vi "FindCircleCenter.vi"(7 "error in":errorcluster) -> (27 "error out":errorcluster)   [LabVIEW 2017]
uses:
  <vilib>/gmath/GlobalOptimization.llb/DE_State.ctl
  <vilib>/gmath/GlobalOptimization.llb/DE_Population.ctl
  <vilib>/vision/NI_Vision_Development_Module.lvlib
  <vilib>/gmath/NI_AAL_GlobalOptimization.lvlib
panel:
  out "Ending State":T1
  out "XY Graph - Dark":cluster{i32[], dbl[]}[](graph) caption="XY Graph - dark"
  out "Image Out":T3(plugin-control)
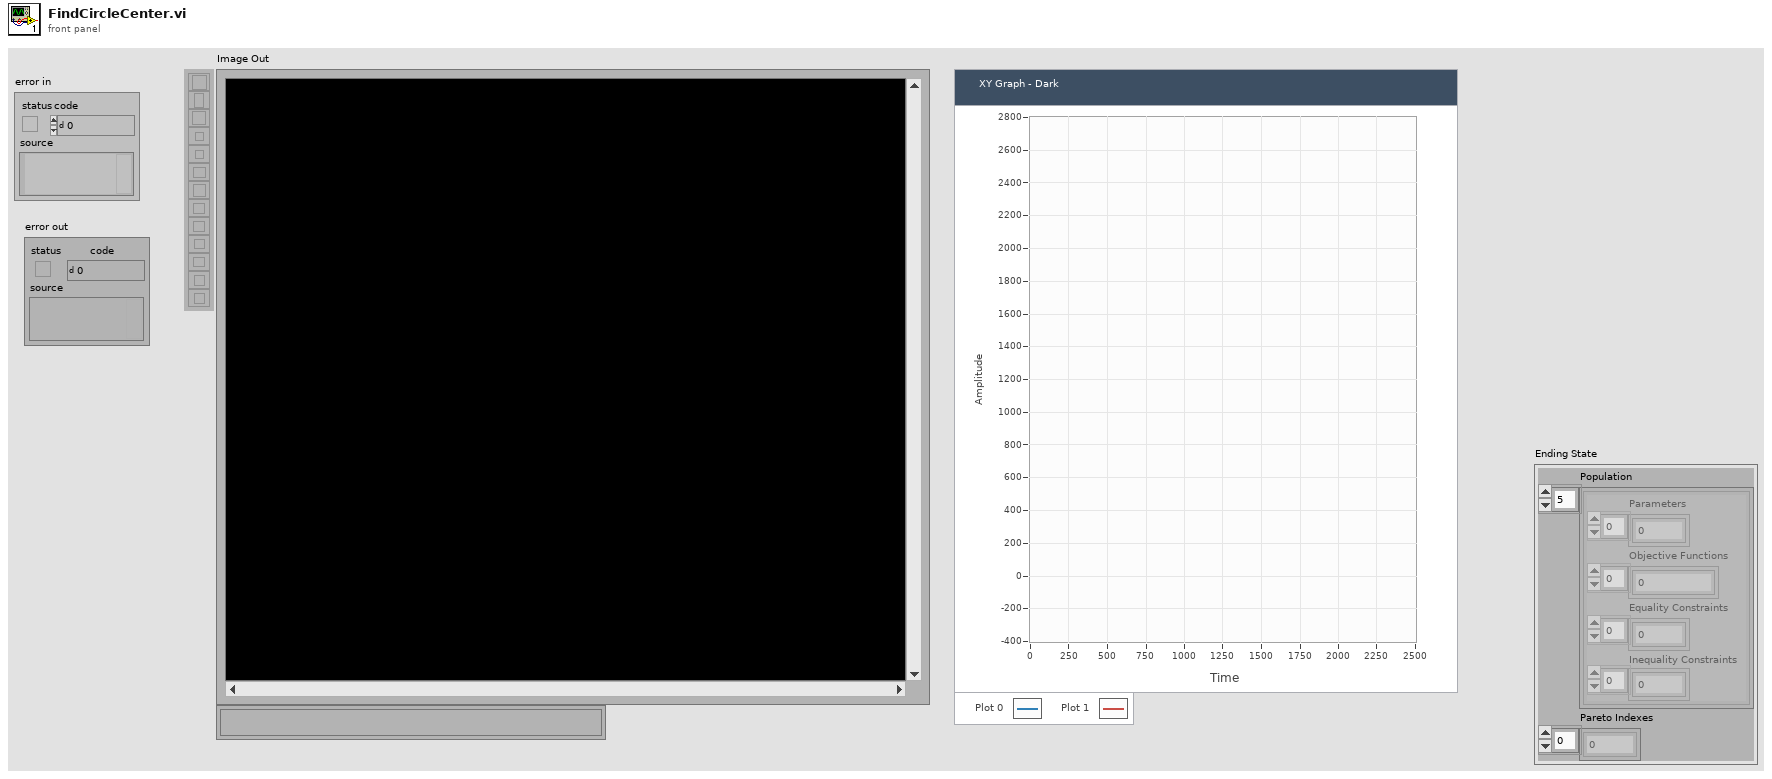
[diagram p1: front panel]
types:
  T1 = typedef "NI_AAL_GlobalOptimization.lvlib/DE_State.ctl" = cluster{"Population":T2[], "Pareto Indexes":i32[]}
  T2 = typedef "NI_AAL_GlobalOptimization.lvlib/DE_Population.ctl" = cluster{"Parameters":dbl[], "Objective Functions":dbl[], "Equality Constraints":dbl[], "Inequality Constraints":dbl[]}
  T3 = typedef "IMAQ Image.ctl" = refnum<image>
  T4 = enum32{"Differentiation", "Gradient", "Prewitt", "Roberts", "Sigma", "Sobel"}
  T5 = typedef "Image Type" = u32
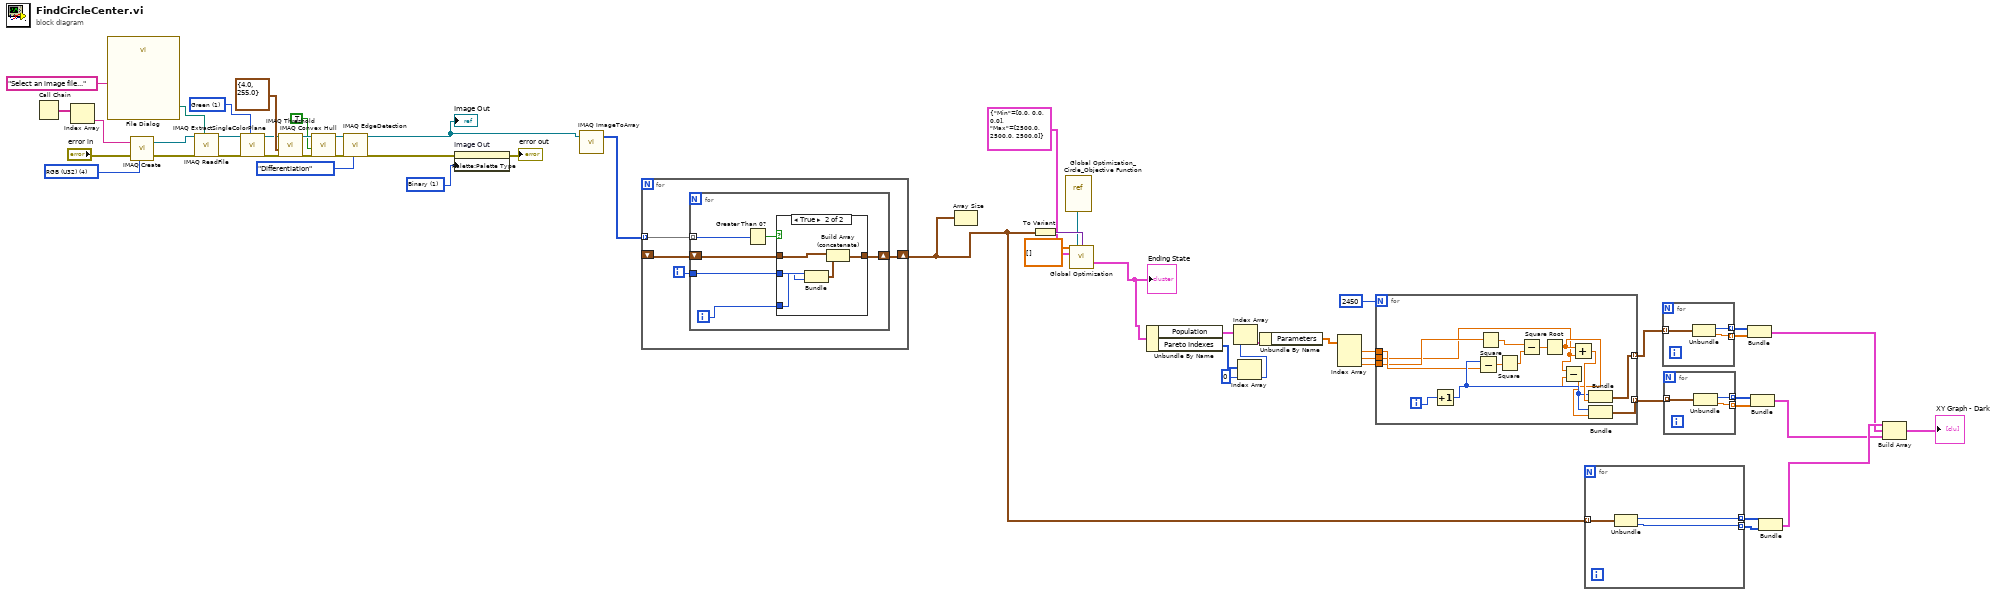
[diagram p0: block diagram]
diagram:
  w31 = u32 1 items=["Grayscale", "Binary", "Gradient", "Rainbow", "Temperature", "User Defined", "Binary 16 Bit", "Gradient 16 Bit", "Rainbow 16 Bit", "Temperature 16 Bit", "User Defined 16 Bit"] ("Palette Type")
  w45 = 1 items=["Red", "Green", "Blue", "Hue", "Saturation", "Luminance", "Value", "Intensity"] ("Color Plane")
  w46 = T5 4 items=["Grayscale (U8)", "Grayscale (I16)", "Grayscale (SGL)", "Complex (CSG)", "RGB (U32)", "HSL (U32)", "RGB (U64)", "Grayscale (U16)"] ("Image Type")
  n1 = Call Chain() -> (call chain=w50:string[])
  n2 = Index Array(array=w50) -> (element=w49:string)  [unwired: 1 in]
  n3 = call "File Dialog"("prompt"="Select an image file...") -> ("selected path"=w47:path)  [unwired: 6 in, 8 out]
  n4 = call "IMAQ Create"("Image Name"=w49, "Image Type"=w46, "error in (no error)"="error in") -> ("New Image"=w53:T3, "error out"=w52:errorcluster)  [unwired: 1 in, 1 out]
  n5 = call "IMAQ ReadFile"("File Path"=w47, "error in (no error)"=w52, "Image"=w53) -> ("error out"=w43:errorcluster, "Image Out"=w44:T3)  [unwired: 2 in, 5 out]
  n6 = call "IMAQ ExtractSingleColorPlane"("Color Plane"=w45, "error in (no error)"=w43, "Image Src"=w44) -> ("error out"=w40:errorcluster, "Image Dst Out"=w41:T3)  [unwired: 1 in, 6 out]
  n7 = call "IMAQ Threshold"("error in (no error)"=w40, "Range"=cluster{"Lower value":sgl, "Upper value":sgl} {"Lower value"=4.0, "Upper value"=255.0}, "Image Src"=w41) -> ("error out"=w38:errorcluster, "Image Dst Out"=w39:T3)  [unwired: 3 in, 4 out]
  n8 = call "IMAQ Convex Hull"("error in (no error)"=w38, "Connectivity 4/8 (8)"=TRUE, "Image Src"=w39) -> ("error out"=w34:errorcluster, "Image Dst Out"=w35:T3)  [unwired: 1 in, 6 out]
  n9 = call "IMAQ EdgeDetection"("Method"=T4."Differentiation", "error in (no error)"=w34, "Image Src"=w35) -> ("error out"=w33:errorcluster, "Image Dst Out"=w30:T3)  [unwired: 3 in, 4 out]
  "Image Out" <- w30
  n10 = property on="Image Out" class="ImageControl"(error in=w33, "Palette:Palette Type"=w31) -> (error out=→"error out":errorcluster)  [unwired: 1 in, 1 out]
  n11 = call "IMAQ ImageToArray"("Image"=w30) -> ("Image Pixels (U8)"=w29:u8[][])  [unwired: 3 in, 4 out]
  n12 = for {
    tunnel: w29 -> [w57] mode=indexing
    shift-right: [w55] -> w22
    shift-left: _ -> [w54]
    i -> [w56]
    n13 = for {
      tunnel: w57 -> [w63] mode=indexing
      tunnel: w56 -> [w61]
      shift-right: [w59] -> w55
      shift-left: w54 -> [w58]
      i -> [w60]
      n14 = Greater Than 0?(x=w63) -> (x > 0?=w62:bool)
      n15 = case shown="True" w62 {
        tunnel: w61 -> [_ w65]
        tunnel: w60 -> [_ w66]
        tunnel: [w64 w68] -> w59
        tunnel: w58 -> [w64 w67]
        frame False {
        }
        frame True {
          n16 = Bundle(w66, w65) -> (w69:cluster{i32, i32})  [unwired: 1 in]
          n17 = Build Array (concatenate)(w67, w69) -> (w68:cluster{i32, i32}[])
        }
      }
    }
  }
  n18 = Array Size(array=w22) -> ()  [unwired: 1 out]
  n19 = To Variant(anything=w22) -> (Variant=w28:variant)
  n20 = vi-ref "Global Optimization_Circle_Objective Function.vi"() -> (w27:refnum<vi>)
  n21 = call <vilib>:"Global Optimization.vi"("Init Parameters"=dbl[][] [], "objective and constraint function"=w27, "function data"=w28, "Bounds"=cluster{"Min":dbl[], "Max":dbl[]} {"Min"=[0.0, 0.0, 0.0], "Max"=[2500.0, 2500.0, 2500.0]}) -> ("Ending State"=w7:T1)  [unwired: 7 in, 4 out]
  "Ending State" <- w7
  n22 = Unbundle By Name(w7) -> ("Population"=w8:T2[], "Pareto Indexes"=w6:i32[])
  n23 = Index Array(array=w6, index=0) -> (element=w5:i32)
  n24 = Index Array(array=w8, index=w5) -> (element=w9:T2)
  n25 = Unbundle By Name(w9) -> ("Parameters"=w10:dbl[])
  n26 = Index Array(array=w10) -> (element #1=w4:dbl, element #2=w3:dbl, element #3=w2:dbl)  [unwired: 3 in]
  n27 = for {
    N: 2450 -> [_]
    tunnel: [w83] -> w19 mode=indexing
    tunnel: [w73] -> w14 mode=indexing
    tunnel: w4 -> [w72]
    tunnel: w3 -> [w70]
    tunnel: w2 -> [w71]
    i -> [w82]
    n28 = Increment(x=w82) -> (x+1=w76:i32)
    n29 = Subtract(x=w76, y=w72) -> (x-y=w81:dbl)
    n30 = Square(x=w71) -> (x^2=w80:dbl)
    n31 = Square(x=w81) -> (x^2=w79:dbl)
    n32 = Subtract(x=w80, y=w79) -> (x-y=w78:dbl)
    n33 = Square Root(x=w78) -> (sqrt(x)=w75:dbl)
    n34 = Subtract(x=w70, y=w75) -> (x-y=w74:dbl)
    n35 = Add(x=w75, y=w70) -> (x+y=w77:dbl)
    n36 = Bundle(w76, w77) -> (w83:cluster{i32, dbl})  [unwired: 1 in]
    n37 = Bundle(w76, w74) -> (w73:cluster{i32, dbl})  [unwired: 1 in]
  }
  n38 = for {
    tunnel: w22 -> [w86] mode=indexing
    tunnel: [w85] -> w21 mode=indexing
    tunnel: [w84] -> w20 mode=indexing
    n39 = Unbundle(w86) -> (w85:i32, w84:i32)
  }
  n40 = for {
    tunnel: w19 -> [w89] mode=indexing
    tunnel: [w88] -> w18 mode=indexing
    tunnel: [w87] -> w17 mode=indexing
    n41 = Unbundle(w89) -> (w88:i32, w87:dbl)
  }
  n42 = for {
    tunnel: w14 -> [w92] mode=indexing
    tunnel: [w91] -> w13 mode=indexing
    tunnel: [w90] -> w12 mode=indexing
    n43 = Unbundle(w92) -> (w91:i32, w90:dbl)
  }
  n44 = Bundle(w18, w17) -> (w15:cluster{i32[], dbl[]})  [unwired: 1 in]
  n45 = Bundle(w13, w12) -> (w11:cluster{i32[], dbl[]})  [unwired: 1 in]
  n46 = Bundle(w21, w20) -> (w16:cluster{i32[], i32[]})  [unwired: 1 in]
  n47 = Build Array(w16, w15, w11) -> (→"XY Graph - Dark":cluster{i32[], dbl[]}[])
